vi "플랜b.vi"   [LabVIEW 2015]
uses:
  <vilib>/NXT/Subs/MotorOutput.ctl
  <vilib>/NXT/Block Support/NXT_InputPort.ctl
  <vilib>/NXT/Dual Mode Library/Sensors/Light_On.vi
  <vilib>/NXT/Dual Mode Library/Motors/MotorReverse.vi
  <vilib>/NXT/Dual Mode Library/Waits/Wait_Num.vi
  <vilib>/NXT/Dual Mode Library/Motors/MotorOn.vi
  <vilib>/NXT/Dual Mode Library/Sensors/Sonar_cm.vi
types:
  T1 = typedef "NXT_InputPort.ctl" = u32
  T2 = typedef "MotorOutput.ctl" = u8
  T3 = typedef "LVHSConnector.ctl" = refnum<class "BrickReference.lvclass">
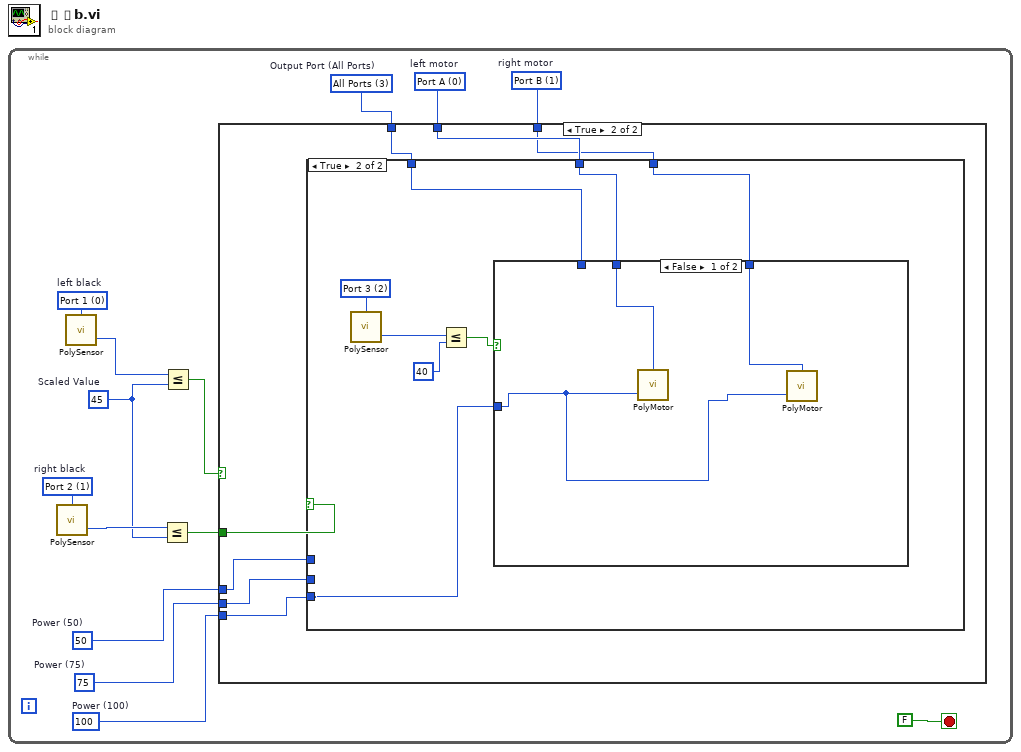
[diagram p0: block diagram]
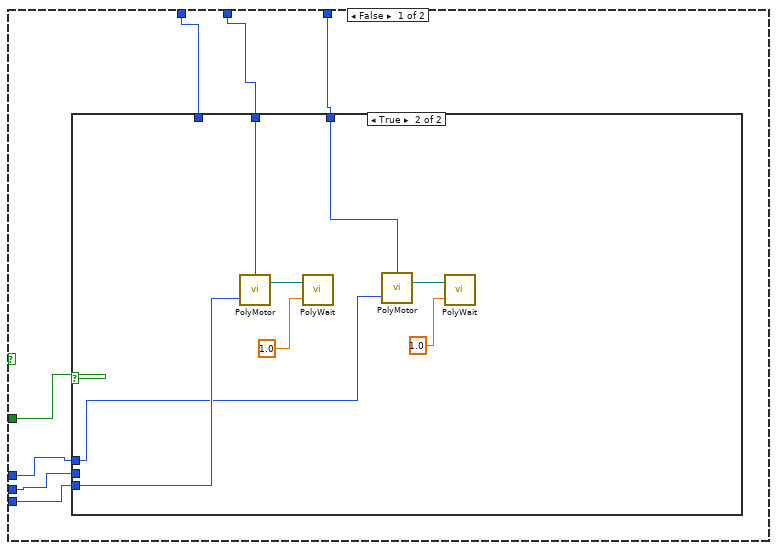
[diagram p2: hidden frame]
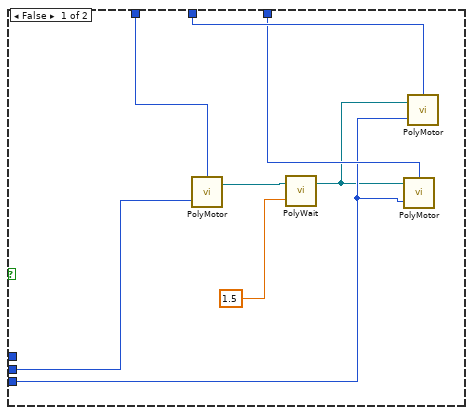
[diagram p3: hidden frame]
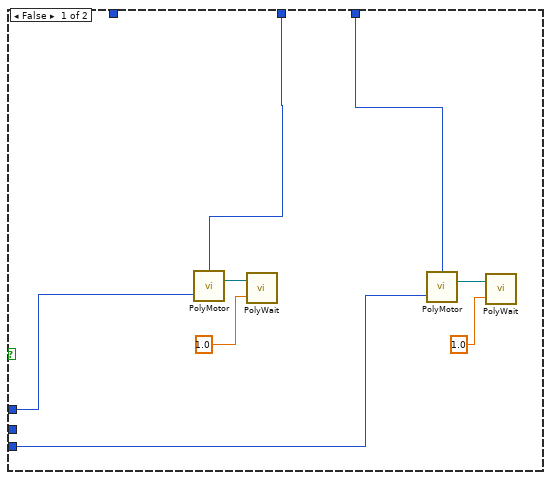
[diagram p4: hidden frame]
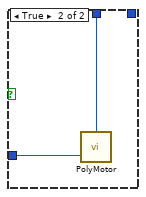
[diagram p5: hidden frame]
diagram:
  n1 = while {
    stop <- FALSE ("stop") stop-if-true
    w4 = 100  # Power (100)
    w8 = 75  # Power (75)
    w3 = 50  # Power (50)
    w9 = T1 1 items=["Port 1", "Port 2", "Port 3", "Port 4"]  # right black
    w12 = T1 0 items=["Port 1", "Port 2", "Port 3", "Port 4"]  # left black
    w6 = T2 1 items=["Port A"=0, "Port B"=1, "Port C"=2, "Ports A & B"=4, "Ports A & C"=5, "Ports B & C"=6, "All Ports"=3]  # right motor
    w5 = T2 0 items=["Port A"=0, "Port B"=1, "Port C"=2, "Ports A & B"=4, "Ports A & C"=5, "Ports B & C"=6, "All Ports"=3]  # left motor
    w13 = T2 3 items=["Port A"=0, "Port B"=1, "Port C"=2, "Ports A & B"=4, "Ports A & C"=5, "Ports B & C"=6, "All Ports"=3]  # Output Port (All Ports)
    w1 = i16 45  # Scaled Value
    n2 = call-poly <vilib>:"PolySensor.vi"("Port (Port 3)"=w9) -> ("Scaled Value"=w10:i16)  [unwired: 2 in, 1 out]
    n3 = call-poly <vilib>:"PolySensor.vi"("Port (Port 3)"=w12) -> ("Scaled Value"=w11:i16)  [unwired: 2 in, 1 out]
    n4 = Less Or Equal?(x=w10, y=w1) -> (x <= y?=w7:bool)
    n5 = Less Or Equal?(x=w11, y=w1) -> (x <= y?=w2:bool)
    n6 = case shown="True" w2 {
      tunnel: w13 -> [w20 w43]
      tunnel: w8 -> [w18 w40]
      tunnel: w7 -> [w21 w44]
      tunnel: w6 -> [w19 w41]
      tunnel: w5 -> [w15 w42]
      tunnel: w4 -> [w17 w39]
      tunnel: w3 -> [w16 w38]
      frame False {
        n7 = case shown="True" w21 {
          tunnel: w20 -> [w29 _]
          tunnel: w18 -> [w28 _]
          tunnel: w15 -> [w25 w33]
          tunnel: w19 -> [w24 w32]
          tunnel: w17 -> [w23 w31]
          tunnel: w16 -> [_ w30]
          frame False {
            n8 = call-poly <vilib>:"PolyMotor.vi"("Power (75)"=w28, "Output Port (All Ports)"=w29) -> ("NXT/EV3"=w26:T3)  [unwired: 1 in, 1 out]
            n9 = call-poly <vilib>:"PolyWait.vi"("Time (1 sec)"=sgl 1.5, "NXT/EV3"=w26) -> ("NXT/EV3"=w22:T3)  [unwired: 2 in]
            n10 = call-poly <vilib>:"PolyMotor.vi"("Power (75)"=w23, "NXT/EV3"=w22, "Output Port (All Ports)"=w24) -> ()  [unwired: 2 out]
            n11 = call-poly <vilib>:"PolyMotor.vi"("Power (75)"=w23, "NXT/EV3"=w22, "Output Port (All Ports)"=w25) -> ()  [unwired: 2 out]
          }
          frame True {
            n12 = call-poly <vilib>:"PolyMotor.vi"("Power (75)"=w31, "Output Port (All Ports)"=w33) -> ("NXT/EV3"=w37:T3)  [unwired: 1 in, 1 out]
            n13 = call-poly <vilib>:"PolyWait.vi"("Time (1 sec)"=sgl 1.0, "NXT/EV3"=w37) -> ()  [unwired: 2 in, 1 out]
            n14 = call-poly <vilib>:"PolyMotor.vi"("Power (75)"=w30, "Output Port (All Ports)"=w32) -> ("NXT/EV3"=w35:T3)  [unwired: 1 in, 1 out]
            n15 = call-poly <vilib>:"PolyWait.vi"("Time (1 sec)"=sgl 1.0, "NXT/EV3"=w35) -> ()  [unwired: 2 in, 1 out]
          }
        }
      }
      frame True {
        n16 = case shown="True" w44 {
          tunnel: w43 -> [_ w60]
          tunnel: w40 -> [_ _]
          tunnel: w42 -> [w47 w54]
          tunnel: w41 -> [w48 w53]
          tunnel: w39 -> [w45 w59]
          tunnel: w38 -> [w46 _]
          frame False {
            n17 = call-poly <vilib>:"PolyMotor.vi"("Power (75)"=w46, "Output Port (All Ports)"=w47) -> ("NXT/EV3"=w52:T3)  [unwired: 1 in, 1 out]
            n18 = call-poly <vilib>:"PolyWait.vi"("Time (1 sec)"=sgl 1.0, "NXT/EV3"=w52) -> ()  [unwired: 2 in, 1 out]
            n19 = call-poly <vilib>:"PolyMotor.vi"("Power (75)"=w45, "Output Port (All Ports)"=w48) -> ("NXT/EV3"=w51:T3)  [unwired: 1 in, 1 out]
            n20 = call-poly <vilib>:"PolyWait.vi"("Time (1 sec)"=sgl 1.0, "NXT/EV3"=w51) -> ()  [unwired: 2 in, 1 out]
          }
          frame True {
            w56 = T1 2 items=["Port 1", "Port 2", "Port 3", "Port 4"]
            n21 = call-poly <vilib>:"PolySensor.vi"("Port (Port 4)"=w56) -> ("Distance (cm)"=w57:i16)  [unwired: 2 in, 1 out]
            n22 = Less Or Equal?(x=w57, y=i16 40) -> (x <= y?=w55:bool)
            n23 = case shown="False" w55 {
              tunnel: w60 -> [_ w65]
              tunnel: w59 -> [w61 w64]
              tunnel: w54 -> [w63 _]
              tunnel: w53 -> [w62 _]
              frame False {
                n24 = call-poly <vilib>:"PolyMotor.vi"("Power (75)"=w61, "Output Port (All Ports)"=w63) -> ()  [unwired: 1 in, 2 out]
                n25 = call-poly <vilib>:"PolyMotor.vi"("Power (75)"=w61, "Output Port (All Ports)"=w62) -> ()  [unwired: 1 in, 2 out]
              }
              frame True {
                n26 = call-poly <vilib>:"PolyMotor.vi"("Power (75)"=w64, "Output Port (All Ports)"=w65) -> ()  [unwired: 1 in, 2 out]
              }
            }
          }
        }
      }
    }
  }
